vi "Get NVMEM Bytes.vi"(0 "session in":refnum<k21>, 5 "NVMEM area":refnum<k21>="$DefaultNVMEMAreas", 7 "data address":u32 format="%.0x", 9 "data size":u32, 11 "error in (no error)":errorcluster) -> (4 "session out":refnum<k21>, 6 "NVMEM area out":refnum<k21>, 8 "next data address":u32 format="%.0x", 10 "data out":u8[](array[numeric]) format="%.0x", 15 "error out":errorcluster)   [LabVIEW 2020, in "SLSC.lvlib"]
doc: "Reads the specified number of bytes (<B>data size</B>) starting at the given <B>data address</B> in the specified <B>NVMEM area</B>."
uses:
  <vilib>/SLSC/SLSC.lvlib
  nislsclvapi.dll
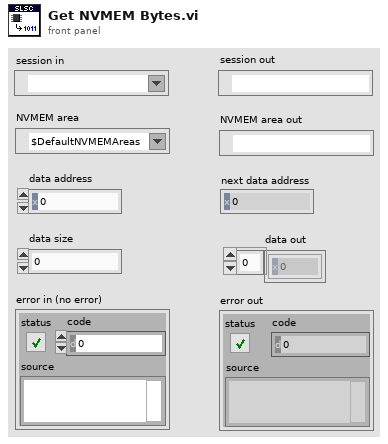
[diagram p1: front panel]
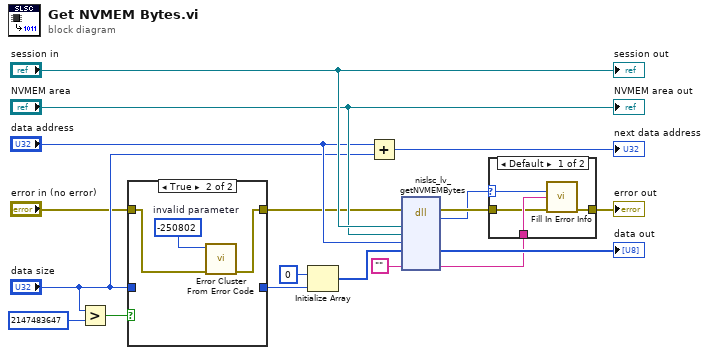
[diagram p0: block diagram]
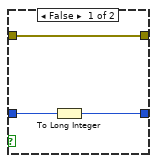
[diagram p2: hidden frame]
diagram:
  n1 = Greater?(x="data size", y=u32 2147483647) -> (0:w3:bool)
  n2 = case shown="True" w3 {
    tunnel: [w21 _] -> w6
    tunnel: "data size" -> [w20 _]
    tunnel: "error in (no error)" -> [w19 w24]
    tunnel: [w19 w23] -> w1
    frame False {
      n3 = To Long Integer(number=w20) -> (32bit integer=w21:i32)
    }
    frame True {
      w22 = -250802  # invalid parameter
      n4 = call <vilib>:"Error Cluster From Error Code.vi"("error in (no error)"=w24, "error code (0)"=w22) -> ("error out"=w23:errorcluster)  [unwired: 7 in]
    }
  }
  n5 = Initialize Array(u8 0, w6) -> (w10:u8[])
  n6 = Add(x="data address", y="data size") -> (x+y=→"next data address":u32)
  n7 = dll-call lib="nislsclvapi.*" fn="nislsc_lv_getNVMEMBytes"(error in=w1, "session"="session in", "nvmemArea"="NVMEM area", "dataAddress"="data address", "data"=w10, "extendedErrorInfo"="") -> (error out=w14:errorcluster, "return type"=w13:i32, "data"=→"data out":u8[], "extendedErrorInfo"=w15:string)  [unwired: 7 in, 1 out]
  n8 = case shown="Default" w13 {
    selector: w13 -> [w28 _]
    tunnel: w15 -> [w27 _]
    tunnel: w14 -> [w26 w29]
    tunnel: [w25 w29] -> w12
    frame Default {
      n9 = call <vilib>:"Fill In Error Info.vi"("status code"=w28, "extended error info"=w27, "error in"=w26) -> ("error out"=w25:errorcluster)  [unwired: 12 in]
    }
    frame 0 {
    }
  }
  "error out" <- w12
  "session out" <- "session in"
  "NVMEM area out" <- "NVMEM area"
